vi "Reset.vi"(0 "VISA resource name":refnum<visa-resource-name>, 1 "Reset to Default (False)":bool, 11 "error in (no error)":errorcluster) -> (4 "VISA resource name out":refnum<visa-resource-name>, 15 "error out":errorcluster)   [LabVIEW 2012, in "Lake Shore Cryotronics 370.lvlib"]
doc: "This VI resets the instrument, and then sends a set of default setup commands to the instrument. \n\nNOTE: If you do not want the instrument reset to its default setup state you MUST set the Reset Defaults control to FALSE."
uses:
  <instrlib>/Lake Shore Cryotronics 370/Lake Shore Cryotronics 370.lvlib
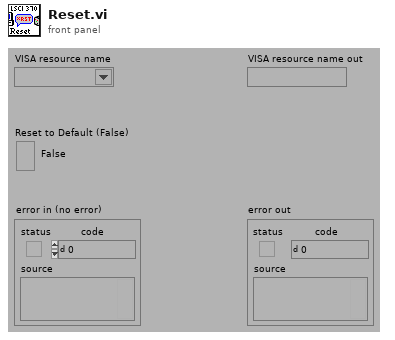
[diagram p1: front panel]
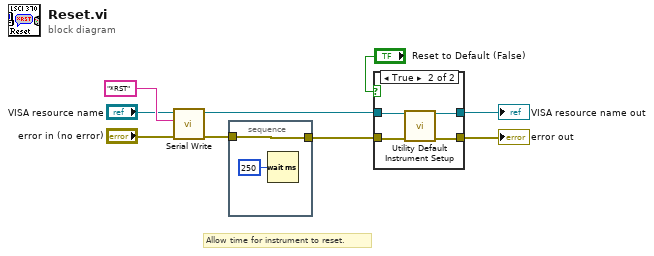
[diagram p0: block diagram]
diagram:
  # "Allow time for instrument to reset."
  n1 = call <instrlib>:"Serial Write.vi"("error in (no error)"="error in (no error)", "Write Buffer (\"\")"="*RST" ("Reset Command"), "VISA resource name"="VISA resource name") -> ("error out"=w2:errorcluster, "VISA resource name out"=w1:refnum<visa-resource-name>)  [unwired: 6 in, 1 out]
  n2 = stacked-sequence {
    tunnel: w2 -> [w10]
    tunnel: [w10] -> w7
    frame #0 {
      n3 = Wait (ms)(milliseconds to wait=u32 250) -> ()  [unwired: 1 out]
    }
  }
  n4 = case shown="True" "Reset to Default (False)" {
    tunnel: [w12 w15] -> w9
    tunnel: [w13 w14] -> w8
    tunnel: w7 -> [w12 w16]
    tunnel: w1 -> [w13 w17]
    frame False {
    }
    frame True {
      n5 = call <instrlib>:"Utility Default Instrument Setup.vi"("VISA resource name"=w17, "error in (no error)"=w16) -> ("VISA resource name out"=w14:refnum<visa-resource-name>, "error out"=w15:errorcluster)  [unwired: 12 in]
    }
  }
  "error out" <- w9
  "VISA resource name out" <- w8
